vi "set_config_cluster.vi"(8 "error in (no error)":errorcluster, 10 "config cluster variant":variant, 11 "FPGAWrapperAK101022Resonance in":refnum<class "FPGAWrapperAK101022Resonance.lvclass">) -> (0 "error out":errorcluster, 3 "FPGAWrapperAK101022Resonance out":refnum<class "FPGAWrapperAK101022Resonance.lvclass">)   [LabVIEW 2010, in "FPGAWrapperAK101022Resonance.lvclass"]
uses:
  FPGAWrapperAK101022Resonance.lvclass
  FPGAWrapperAK101022Resonance.lvclass/FPGAWrapperAK101022Resonance.ctl
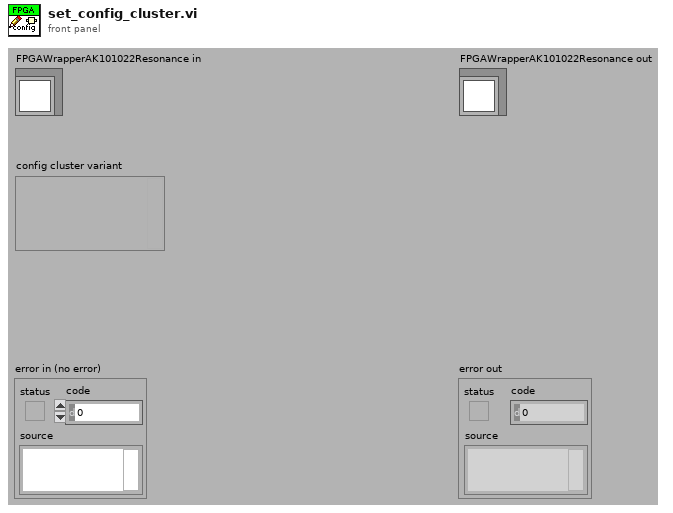
[diagram p1: front panel]
types:
  T1 = typedef "config_data_cluster.ctl" = cluster{"channel offsets":u32[], "invert channel?":bool[]}
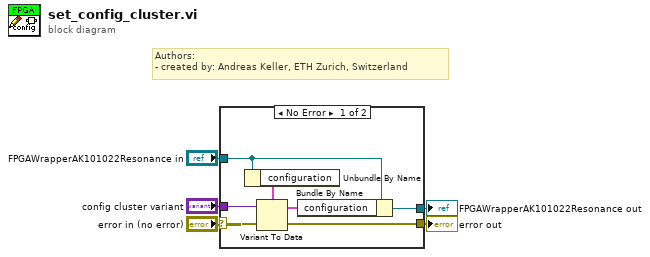
[diagram p0: block diagram]
diagram:
  # "Authors: \n- created by: Andreas Keller, ETH Zurich, Switzerland"
  n1 = case shown="No Error" "error in (no error)" {
    selector: "error in (no error)" -> [w7 w13]
    tunnel: [w6 w13] -> w4
    tunnel: "FPGAWrapperAK101022Resonance in" -> [w9 w14]
    tunnel: "config cluster variant" -> [w12 _]
    tunnel: [w8 w14] -> w1
    frame No Error {
      n2 = Unbundle By Name(w9) -> ("configuration"=w10:T1)
      n3 = Variant To Data(error in=w7, Variant=w12, type=w10) -> (error out=w6:errorcluster, data=w11:T1)
      n4 = Bundle By Name(cluster=w9, "configuration"=w11) -> (w8:refnum<class "FPGAWrapperAK101022Resonance.lvclass">)
    }
    frame Error {
    }
  }
  "error out" <- w4
  "FPGAWrapperAK101022Resonance out" <- w1
